vi "Parse_string.vi"(0 "Input str":string, 1 "PreProcessing":T1, 2 "or string end chars (len is 0)":string, 3 "Desired field (1-n)":u32=1 min=1 step=1, 5 "Data type":T2, 7 "Search Preamble or keyword":string, 9 "Line number (1-n)":u32=1 min=1 step=1, 11 "error in (no error)":errorcluster, 12 "Data qualifier (empty if none)":string, 13 "String length":u32, 14 "Field separator (,)":string=",") -> (4 "Parsed data":string, 6 "Data Valid?":bool, 15 "error out":errorcluster)   [LabVIEW 2013]
uses:
  string_data_type.ctl
  PreProcessStrOp.ctl
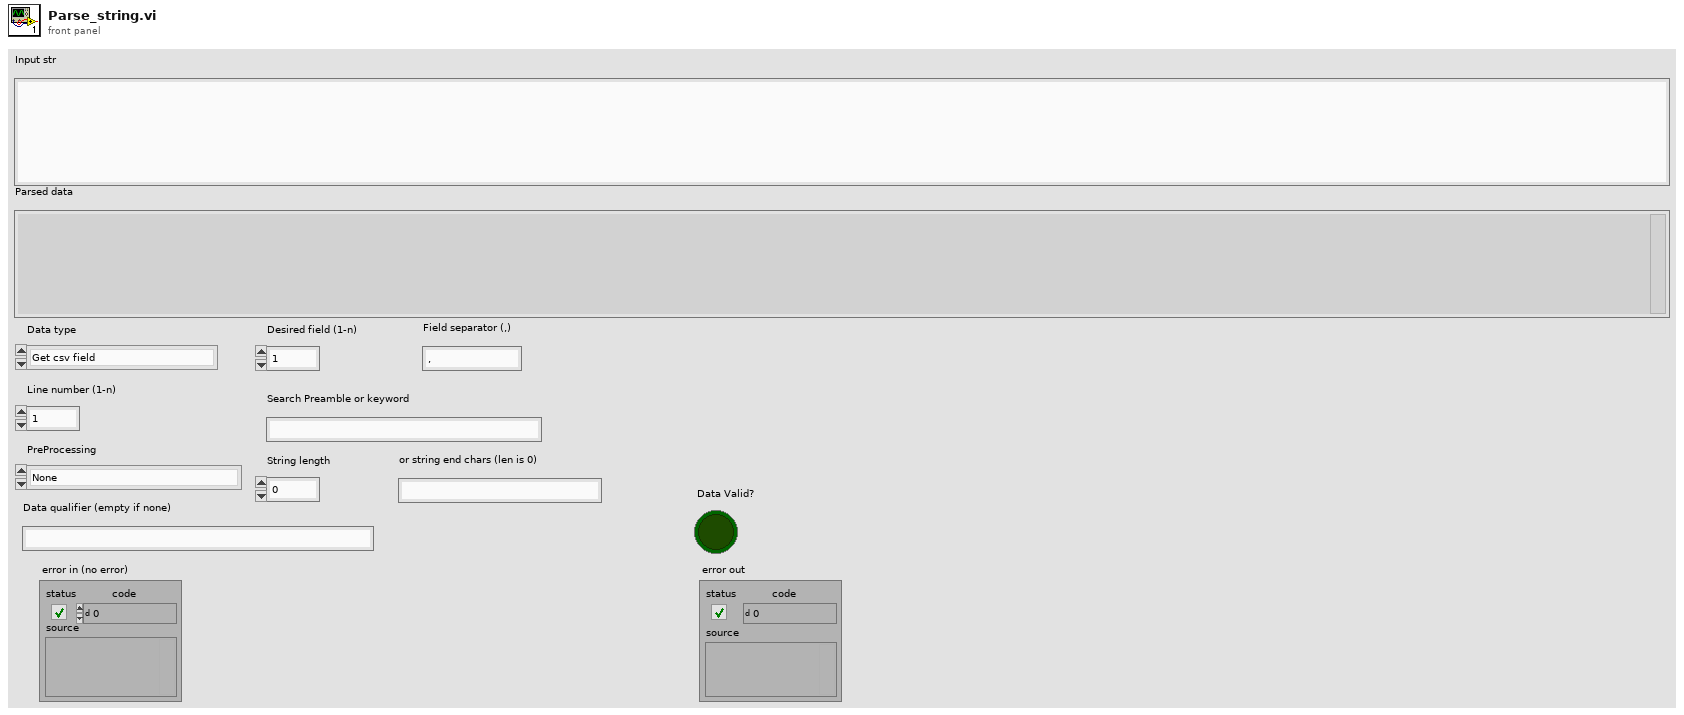
[diagram p1: front panel]
types:
  T1 = typedef "PreProcessStrOp.ctl" = enum16{"None", "Convert to upper case", "Convert to lower case"}
  T2 = typedef "string_data_type.ctl" = enum16{"Get csv field", "Get portion of string", "Get just one line", "Get just one line with keyword", "Just Pre-Process string", "Search and replace", "Search and cut out string"}
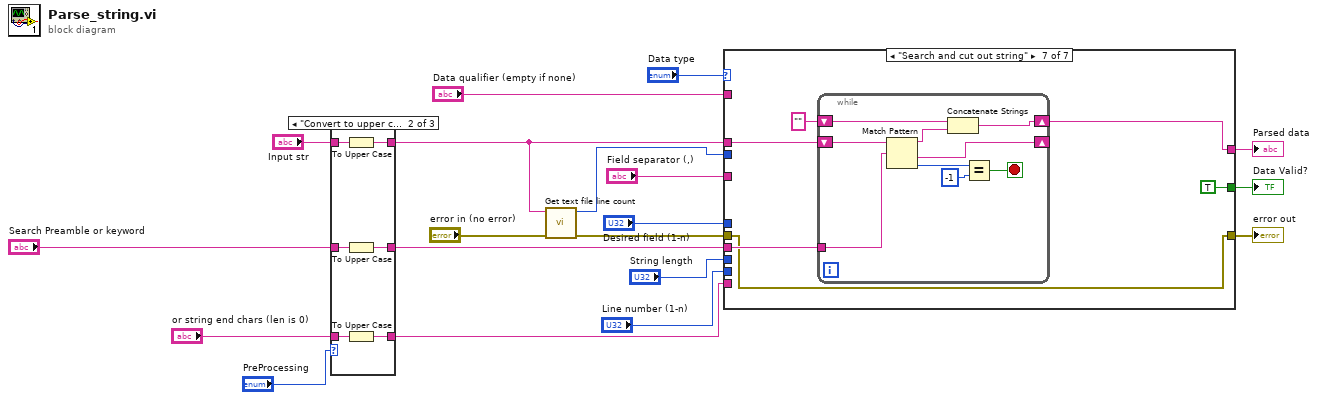
[diagram p0: block diagram]
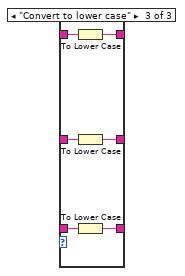
[diagram p3: hidden frame]
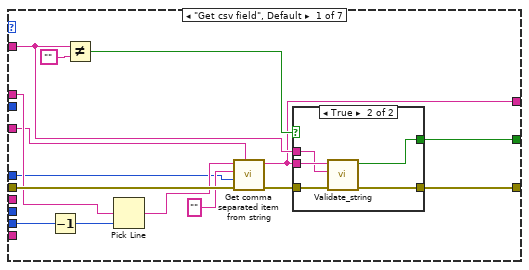
[diagram p4: hidden frame]
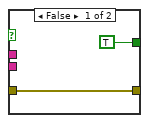
[diagram p5: hidden frame]
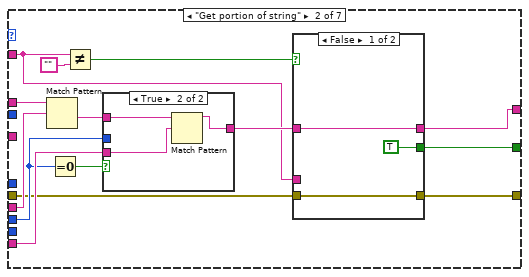
[diagram p6: hidden frame]
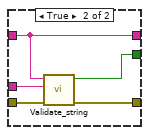
[diagram p7: hidden frame]
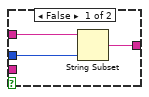
[diagram p8: hidden frame]
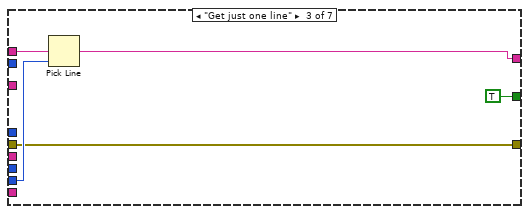
[diagram p9: hidden frame]
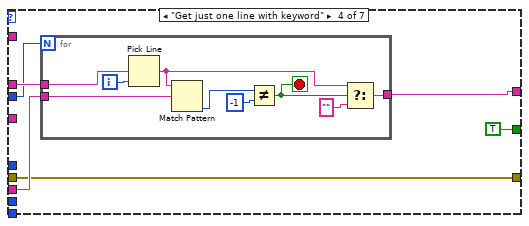
[diagram p10: hidden frame]
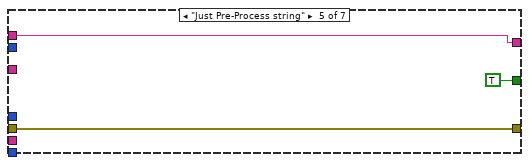
[diagram p11: hidden frame]
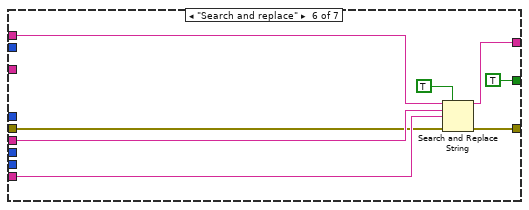
[diagram p12: hidden frame]
diagram:
  n1 = case shown="\"Convert to upper case\"" "PreProcessing" {
    tunnel: "Input str" -> [w22 w28 w34]
    tunnel: [w22 w27 w33] -> w4
    tunnel: "Search Preamble or keyword" -> [w21 w26 w32]
    tunnel: [w21 w25 w31] -> w8
    tunnel: "or string end chars (len is 0)" -> [w20 w23 w29]
    tunnel: [w20 w24 w30] -> w6
    frame "None", Default {
    }
    frame "Convert to upper case" {
      n2 = To Upper Case(1:w28) -> (0:w27:string)
      n3 = To Upper Case(1:w26) -> (0:w25:string)
      n4 = To Upper Case(1:w23) -> (0:w24:string)
    }
    frame "Convert to lower case" {
      n5 = To Lower Case(string=w34) -> (all lower case string=w33:string)
      n6 = To Lower Case(string=w32) -> (all lower case string=w31:string)
      n7 = To Lower Case(string=w29) -> (all lower case string=w30:string)
    }
  }
  n8 = call "Get text file line count.vi"("error in (no error)"="error in (no error)", "Input str"=w4) -> ("error out"=w2:errorcluster, "Lines"=w1:i32)  [unwired: 8 in]
  n9 = case shown="\"Search and cut out string\"" "Data type" {
    tunnel: w2 -> [w49 w61 w85 w91 w105 w110 w117]
    tunnel: "Line number (1-n)" -> [w48 _ w88 _ _ _ _]
    tunnel: w4 -> [w47 w70 w89 w95 w107 w115 w119]
    tunnel: "Desired field (1-n)" -> [w37 _ _ _ _ _ _]
    tunnel: "Data qualifier (empty if none)" -> [w41 w62 _ _ _ _ _]
    tunnel: [w40 w60 w85 w91 w105 w109 w117] -> w15
    tunnel: [w39 w58 w87 w93 w107 w111 w118] -> w14
    tunnel: [w38 w59 TRUE ("String Valid") TRUE ("String Valid") TRUE ("String Valid") TRUE ("String Valid") TRUE ("String Valid")] -> w13
    tunnel: w8 -> [_ w69 _ w94 _ w114 w120]
    tunnel: "String length" -> [_ w65 _ _ _ _ _]
    tunnel: w6 -> [_ w66 _ _ _ w113 _]
    tunnel: "Field separator (,)" -> [w35 _ _ _ _ _ _]
    tunnel: w1 -> [_ _ _ w90 _ _ _]
    frame "Get csv field", Default {
      n10 = Decrement(x=w48) -> (x-1=w44:u32)
      n11 = Not Equal?(x=w41, y="") -> (x != y?=w43:bool)
      n12 = Pick Line(multi-line string=w47, line index=w44) -> (output string=w46:string)  [unwired: 1 in]
      n13 = call "Get comma separated item from string.vi"("Field separator"=w35, "error in (no error)"=w49, "Item number"=w37, "Preamble to first item"="", "String to parse with commas"=w46) -> ("error out"=w42:errorcluster, "Item string value"=w39:string)  [unwired: 5 in]
      n14 = case shown="True" w43 {
        tunnel: w39 -> [_ w56]
        tunnel: w42 -> [w50 w55]
        tunnel: w41 -> [_ w54]
        tunnel: [TRUE ("String Valid") w53] -> w38
        tunnel: [w50 w52] -> w40
        frame False {
        }
        frame True {
          n15 = call "Validate_string.vi"("error in (no error)"=w55, "String data format"=w54, "String"=w56) -> ("error out"=w52:errorcluster, "String Valid"=w53:bool)  [unwired: 7 in]
        }
      }
    }
    frame "Get portion of string" {
      n16 = Match Pattern(string=w70, regular expression=w69) -> (after substring=w67:string)  [unwired: 1 in, 3 out]
      n17 = Equal To 0?(x=w65) -> (x = 0?=w68:bool)
      n18 = Not Equal?(x=w62, y="") -> (x != y?=w64:bool)
      n19 = case shown="True" w68 {
        tunnel: w67 -> [w81 w84]
        tunnel: w66 -> [_ w83]
        tunnel: [w79 w82] -> w63
        tunnel: w65 -> [w80 _]
        frame False {
          n20 = String Subset(string=w81, length (rest)=w80) -> (substring=w79:string)  [unwired: 1 in]
        }
        frame True {
          n21 = Match Pattern(string=w84, regular expression=w83) -> (before substring=w82:string)  [unwired: 1 in, 3 out]
        }
      }
      n22 = case shown="False" w64 {
        tunnel: w63 -> [w71 w74]
        tunnel: w62 -> [_ w78]
        tunnel: w61 -> [w72 w77]
        tunnel: [w72 w76] -> w60
        tunnel: [TRUE ("String Valid") w75] -> w59
        tunnel: [w71 w74] -> w58
        frame False {
        }
        frame True {
          n23 = call "Validate_string.vi"("error in (no error)"=w77, "String data format"=w78, "String"=w74) -> ("error out"=w76:errorcluster, "String Valid"=w75:bool)  [unwired: 7 in]
        }
      }
    }
    frame "Get just one line" {
      n24 = Pick Line(multi-line string=w89, line index=w88) -> (output string=w87:string)  [unwired: 1 in]
    }
    frame "Get just one line with keyword" {
      n25 = for {
        N: w90 -> [_]
        tunnel: w95 -> [w102]
        tunnel: w94 -> [w104]
        tunnel: [w96] -> w93
        i -> [w103]
        stop <- w99 stop-if-true
        n26 = Pick Line(multi-line string=w102, line index=w103) -> (output string=w98:string)  [unwired: 1 in]
        n27 = Match Pattern(string=w98, regular expression=w104) -> (offset past match=w101:i32)  [unwired: 1 in, 3 out]
        n28 = Not Equal?(x=w101, y=-1) -> (x != y?=w99:bool)
        n29 = Select(t=w98, s=w99, f="") -> (s? t:f=w96:string)
      }
    }
    frame "Just Pre-Process string" {
    }
    frame "Search and replace" {
      n30 = Search and Replace String(replace all?=TRUE ("replace all? (F)"), input string=w115, search string=w114, replace string=w113, error in=w110) -> (result string=w111:string, error out=w109:errorcluster)  [unwired: 3 in, 2 out]
    }
    frame "Search and cut out string" {
      n31 = while {
        shift-right: [w123] -> w118
        shift-left: "" -> [w125]
        tunnel: w120 -> [w130]
        shift-right: [w122] -> _
        shift-left: w119 -> [w124]
        stop <- w127 stop-if-true
        n32 = Match Pattern(string=w124, regular expression=w130) -> (before substring=w126:string, after substring=w122:string, offset past match=w129:i32)  [unwired: 1 in, 1 out]
        n33 = Concatenate Strings(w125, w126) -> (w123:string)
        n34 = Equal?(x=w129, y=-1) -> (x = y?=w127:bool)
      }
    }
  }
  "Parsed data" <- w14
  "error out" <- w15
  "Data Valid?" <- w13
